vi "Index Array Elements__ogtk.vi"   [LabVIEW 2016]
doc: "This polymorphic VI returns the <B>elements</B> of a 1D or 2D <B>array</B> at the corresponding <B>indices</B>. For 2D arrays, wire both the <B>indices (row)</B> and <B>indices (col)</B> inputs to specify the row and column of the desired <B>elements</B>."
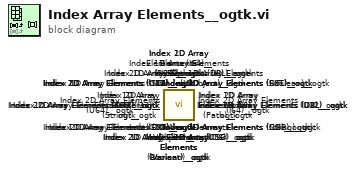
[diagram p0: block diagram]
diagram:
  n1 = call <userlib>:"Index 2D Array Elements (LVObject)__ogtk.vi"() -> ()  [unwired: 11 in, 1 out]
  n2 = call <userlib>:"Index 1D Array Elements (LVObject)__ogtk.vi"() -> ()  [unwired: 11 in, 1 out]
  n3 = call <userlib>:"Index 2D Array Elements (U64)__ogtk.vi"() -> ()  [unwired: 11 in, 1 out]
  n4 = call <userlib>:"Index 2D Array Elements (I64)__ogtk.vi"() -> ()  [unwired: 11 in, 1 out]
  n5 = call <userlib>:"Index 1D Array Elements (U64)__ogtk.vi"() -> ()  [unwired: 11 in, 1 out]
  n6 = call <userlib>:"Index 1D Array Elements (I64)__ogtk.vi"() -> ()  [unwired: 11 in, 1 out]
  n7 = call <userlib>:"Index 1D Array Elements (Boolean)__ogtk.vi"() -> ()  [unwired: 11 in, 1 out]
  n8 = call <userlib>:"Index 1D Array Elements (CDB)__ogtk.vi"() -> ()  [unwired: 11 in, 1 out]
  n9 = call <userlib>:"Index 1D Array Elements (CSG)__ogtk.vi"() -> ()  [unwired: 11 in, 1 out]
  n10 = call <userlib>:"Index 1D Array Elements (CXT)__ogtk.vi"() -> ()  [unwired: 11 in, 1 out]
  n11 = call <userlib>:"Index 1D Array Elements (DBL)__ogtk.vi"() -> ()  [unwired: 11 in, 1 out]
  n12 = call <userlib>:"Index 1D Array Elements (EXT)__ogtk.vi"() -> ()  [unwired: 11 in, 1 out]
  n13 = call <userlib>:"Index 1D Array Elements (I8)__ogtk.vi"() -> ()  [unwired: 11 in, 1 out]
  n14 = call <userlib>:"Index 1D Array Elements (I16)__ogtk.vi"() -> ()  [unwired: 11 in, 1 out]
  n15 = call <userlib>:"Index 1D Array Elements (I32)__ogtk.vi"() -> ()  [unwired: 11 in, 1 out]
  n16 = call <userlib>:"Index 1D Array Elements (Path)__ogtk.vi"() -> ()  [unwired: 11 in, 1 out]
  n17 = call <userlib>:"Index 1D Array Elements (SGL)__ogtk.vi"() -> ()  [unwired: 11 in, 1 out]
  n18 = call <userlib>:"Index 1D Array Elements (String)__ogtk.vi"() -> ()  [unwired: 11 in, 1 out]
  n19 = call <userlib>:"Index 1D Array Elements (U8)__ogtk.vi"() -> ()  [unwired: 11 in, 1 out]
  n20 = call <userlib>:"Index 1D Array Elements (U16)__ogtk.vi"() -> ()  [unwired: 11 in, 1 out]
  n21 = call <userlib>:"Index 1D Array Elements (U32)__ogtk.vi"() -> ()  [unwired: 11 in, 1 out]
  n22 = call <userlib>:"Index 1D Array Elements (Variant)__ogtk.vi"() -> ()  [unwired: 11 in, 1 out]
  n23 = call <userlib>:"Index 2D Array Elements (Boolean)__ogtk.vi"() -> ()  [unwired: 11 in, 1 out]
  n24 = call <userlib>:"Index 2D Array Elements (CDB)__ogtk.vi"() -> ()  [unwired: 11 in, 1 out]
  n25 = call <userlib>:"Index 2D Array Elements (CSG)__ogtk.vi"() -> ()  [unwired: 11 in, 1 out]
  n26 = call <userlib>:"Index 2D Array Elements (CXT)__ogtk.vi"() -> ()  [unwired: 11 in, 1 out]
  n27 = call <userlib>:"Index 2D Array Elements (DBL)__ogtk.vi"() -> ()  [unwired: 11 in, 1 out]
  n28 = call <userlib>:"Index 2D Array Elements (EXT)__ogtk.vi"() -> ()  [unwired: 11 in, 1 out]
  n29 = call <userlib>:"Index 2D Array Elements (I8)__ogtk.vi"() -> ()  [unwired: 11 in, 1 out]
  n30 = call <userlib>:"Index 2D Array Elements (I16)__ogtk.vi"() -> ()  [unwired: 11 in, 1 out]
  n31 = call <userlib>:"Index 2D Array Elements (I32)__ogtk.vi"() -> ()  [unwired: 11 in, 1 out]
  n32 = call <userlib>:"Index 2D Array Elements (Path)__ogtk.vi"() -> ()  [unwired: 11 in, 1 out]
  n33 = call <userlib>:"Index 2D Array Elements (SGL)__ogtk.vi"() -> ()  [unwired: 11 in, 1 out]
  n34 = call <userlib>:"Index 2D Array Elements (String)__ogtk.vi"() -> ()  [unwired: 11 in, 1 out]
  n35 = call <userlib>:"Index 2D Array Elements (U8)__ogtk.vi"() -> ()  [unwired: 11 in, 1 out]
  n36 = call <userlib>:"Index 2D Array Elements (U16)__ogtk.vi"() -> ()  [unwired: 11 in, 1 out]
  n37 = call <userlib>:"Index 2D Array Elements (U32)__ogtk.vi"() -> ()  [unwired: 11 in, 1 out]
  n38 = call <userlib>:"Index 2D Array Elements (Variant)__ogtk.vi"() -> ()  [unwired: 11 in, 1 out]
